vi "Compute Arbitrary Signal Reference.vi"(0 "Level in":refnum<class "Level.lvclass">, 7 "signal":dbl[](array[numeric]), 9 "Fs":dbl, 11 "error in (no error)":errorcluster) -> (4 "Level out":refnum<class "Level.lvclass">, 8 "ref":dbl, 15 "error out":errorcluster)   [LabVIEW 2020, in "Level.lvclass"]
uses:
  Level.lvclass
  Level.lvclass/Level.ctl
  432b65f3-da21-4b4e-85d8-e4efab7ed184.vi
  Utility VIs/Math VIs/FFT x(t) to dB,Degrees (1D).vi
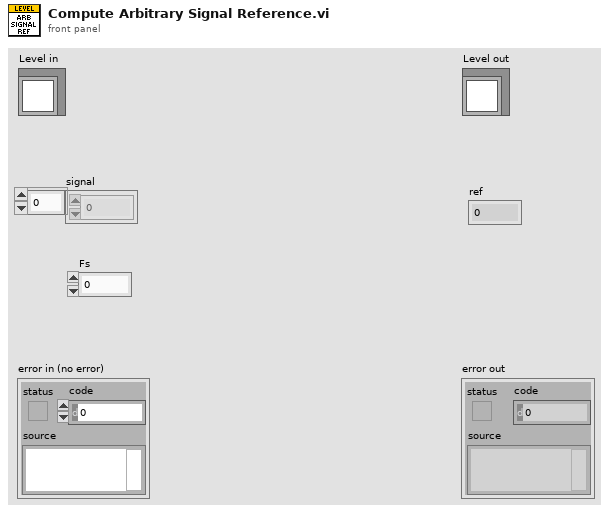
[diagram p1: front panel]
types:
  T1 = typedef "Level.lvclass/LevelUnits.ctl" = enum16{"dB atten", "dB SPL", "dB Vrms", "Volts", "dB mW", "mW", "dB HL", "dB SL"}
  T2 = cluster{"Freq (Hz)":dbl[], "Mag (dB SPL)":dbl[], "Phase (deg)":dbl[]}
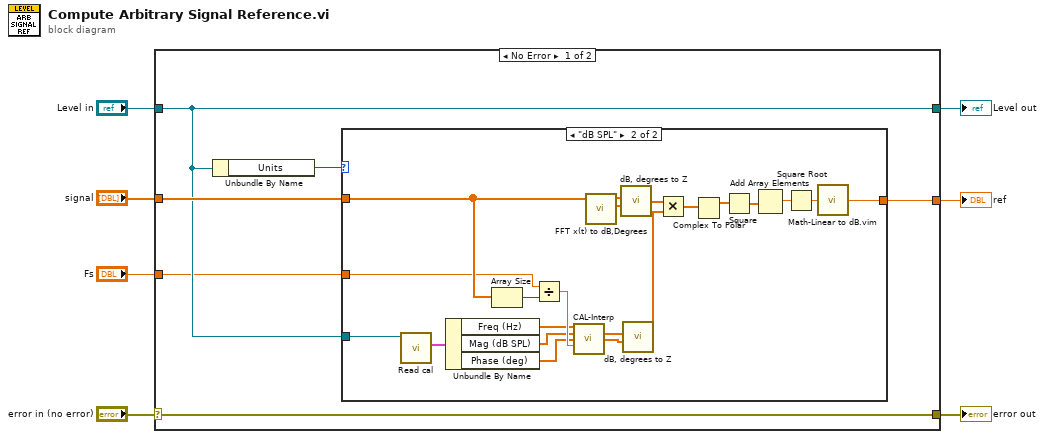
[diagram p0: block diagram]
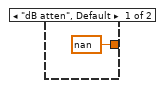
[diagram p2: hidden frame]
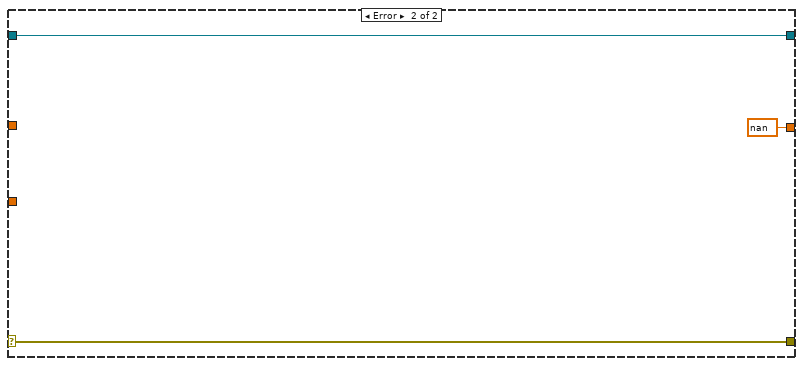
[diagram p3: hidden frame]
diagram:
  n1 = case shown="No Error" "error in (no error)" {
    selector: "error in (no error)" -> [w13 w38]
    tunnel: [w13 w38] -> w6
    tunnel: [w10 w37] -> w4
    tunnel: "Level in" -> [w10 w37]
    tunnel: "signal" -> [w11 _]
    tunnel: "Fs" -> [w9 _]
    tunnel: [w8 nan ("dB")] -> w1
    frame No Error {
      n2 = Unbundle By Name(w10) -> ("Units"=w12:T1)
      n3 = case shown="\"dB SPL\"" w12 {
        tunnel: w11 -> [_ w17]
        tunnel: w10 -> [_ w18]
        tunnel: w9 -> [_ w16]
        tunnel: [nan ("dB") w15] -> w8
        frame "dB atten", Default {
        }
        frame "dB SPL" {
          n4 = call "Read cal.vi"("Level in"=w18) -> ("cal"=w30:T2)  [unwired: 8 in, 2 out]
          n5 = Unbundle By Name(w30) -> ("Freq (Hz)"=w31:dbl[], "Mag (dB SPL)"=w32:dbl[], "Phase (deg)"=w33:dbl[])
          n6 = Array Size(array=w17) -> (size(s)=w34:i32)
          n7 = Divide(x=w16, y=w34) -> (x/y=w35:dbl)
          n8 = call "CAL-Interp.vi"("Frequency (Hz)"=w31, "Magnitude (dB)"=w32, "Phase (degrees)"=w33, "df (Hz)"=w35) -> ("Interp Magnitude (dB)"=w28:dbl[], "Interp Phase (degrees)"=w27:dbl[])  [unwired: 8 in, 2 out]
          n9 = call-poly "FFT x(t) to dB,Degrees.vi"("X"=w17) -> ("+Freq Phase of FFT (degrees)"=w25:dbl[], "+Freq. Mag of FFT (dB rms)"=w26:dbl[])  [unwired: 8 in, 1 out]
          n10 = call "dB, degrees to Z.vi"("Magnitude (dB)"=w26, "Phase (degrees)"=w25) -> ("Z"=w20:cdb[])  [unwired: 5 in]
          n11 = call "dB, degrees to Z.vi"("Magnitude (dB)"=w28, "Phase (degrees)"=w27) -> ("Z"=w29:cdb[])  [unwired: 5 in]
          n12 = Multiply(x=w20, y=w29) -> (x*y=w19:cdb[])
          n13 = Complex To Polar(r * e^(i*theta)=w19) -> (r=w21:dbl[])  [unwired: 1 out]
          n14 = Square(x=w21) -> (x^2=w24:dbl[])
          n15 = Add Array Elements(numeric array=w24) -> (sum=w23:dbl)
          n16 = Square Root(x=w23) -> (sqrt(x)=w22:dbl)
          n17 = call "Math-Linear to dB.vim"("linear"=w22) -> ("dB"=w15:dbl)
        }
      }
    }
    frame Error {
    }
  }
  "error out" <- w6
  "Level out" <- w4
  "ref" <- w1
